vi "send8bit UINT Volume Data To Sink.vi"(4 "pDepthInVoxels":i32, 5 "pHeightInVoxels":i32, 6 "pWidthInVoxels":i32, 7 "pBufferLength":i64, 9 "pBufferAddress":string, 10 "pChannelId":i32, 11 "pSinkId":i32) -> (1 "pBufferAddress out":string, 3 "function return":i32)   [LabVIEW 2012, in "cvlib.lvlib"]
doc: "extern \"C\" __declspec(dllexport) long __cdecl send8bitUINTVolumeDataToSink( long pSinkId,\n long pChannelId,\n char *pBufferAddress,\n __int64 pBufferLength,\n long pWidthInVoxels,\n long pHeightInVoxels,\n long pDepthInVoxels);"
uses:
  cvlib.lvlib
  cvlib.dll
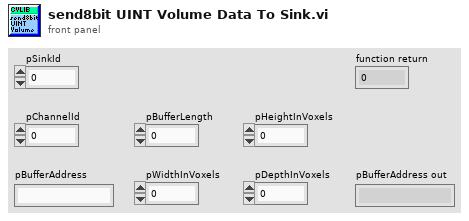
[diagram p1: front panel]
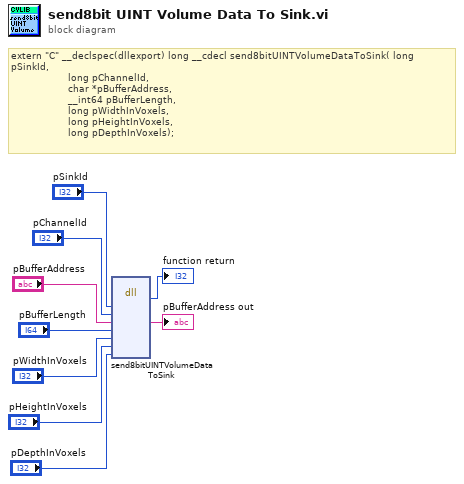
[diagram p0: block diagram]
diagram:
  # "extern \"C\" __declspec(dllexport) long __cdecl send8bitUINTVolumeDataToSink( long pSinkId,\n\t\t\t\t\t\t\t\t\t\t\t\t\t\t\t\t\t\t\tlong pChannelId,\n\t\t\t\t\t\t\t\t\t\t\t\t\t\t\t\t\t\t\tchar *pBufferAddress,\n\t\t\t\t\t\t\t\t\t\t\t\t\t\t\t\t\t\t\t__int64 pBufferLength,\n\t\t\t\t\t\t\t\t\t\t\t\t\t\t\t\t\t\t\tlong pWidthInVoxels,\n\t\t\t\t\t\t\t\t\t\t\t\t\t\t\t\t\t\t\tlong pHeightInVoxels,\n\t\t\t\t\t\t\t\t\t\t\t\t\t\t\t\t\t\t\tlong pDepthInVoxels);"
  n1 = dll-call lib="C:/Users/myerslab/workspace2/Libraries/ClearVolume/cpp/labview/lvcvlib/cvlib.*" fn="send8bitUINTVolumeDataToSink"("pSinkId"="pSinkId", "pChannelId"="pChannelId", "pBufferAddress"="pBufferAddress", "pBufferLength"="pBufferLength", "pWidthInVoxels"="pWidthInVoxels", "pHeightInVoxels"="pHeightInVoxels", "pDepthInVoxels"="pDepthInVoxels") -> (→"function return":i32, "pBufferAddress"=→"pBufferAddress out":string)  [unwired: 9 in, 2 out]
